vi "file.close.vi"(8 "error in":errorcluster, 11 "midi-file in":refnum<class "midi-file.lvclass">) -> (0 "error out":errorcluster)   [LabVIEW 2020, in "midi-file.lvclass"]
uses:
  midi-file.lvclass
  midi-file.lvclass/midi-file.ctl
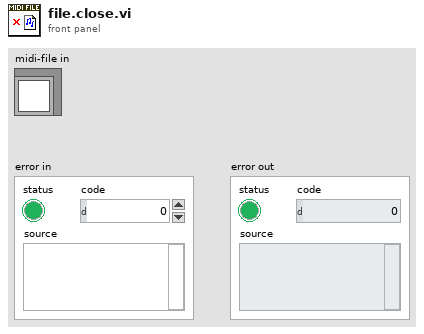
[diagram p1: front panel]
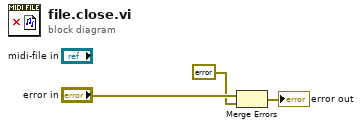
[diagram p0: block diagram]
diagram:
  n1 = Merge Errors("error in", errorcluster {"status"=FALSE, "code"=0, "source"=""} ("error in")) -> (→"error out":errorcluster)
